vi "Count Encoder Advanced.vi"(6 "Initialise":bool, 7 "Filter Iterations":i16=2, 9 "Encoder B Signal In":bool, 10 "Encoder A Signal In":bool) -> (1 "dt (uS)":i64, 2 "Encoder Count Out":i64)   [LabVIEW 2014]
uses:
  <vilib>/rvi/Emulation/niFpgaGetClockAttributes.vi
  <vilib>/rvi/Emulation/niFpgaSctlEmulationGetInTimedLoop.vi
  <vilib>/rvi/Emulation/niFpgaEmulationReportErrorSimple.vi
  <vilib>/rvi/Emulation/niFpgaCriticalErrorInLSC.vi
panel:
  # "Inputs"
  # "Outputs"
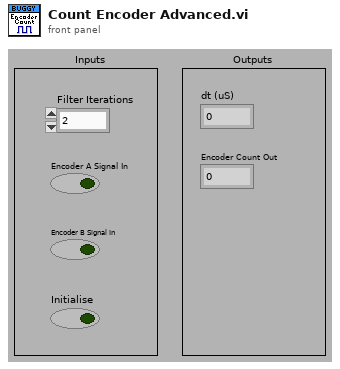
[diagram p1: front panel]
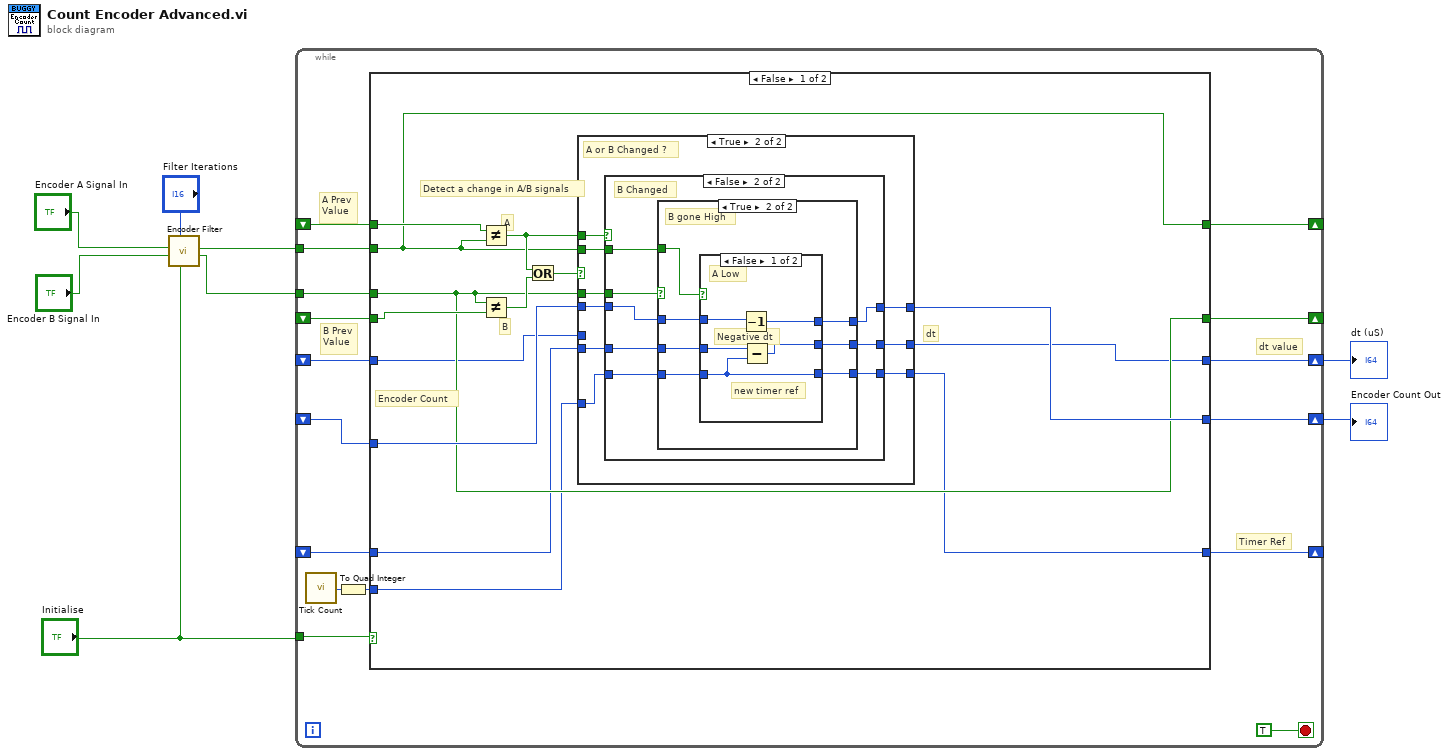
[diagram p0: block diagram]
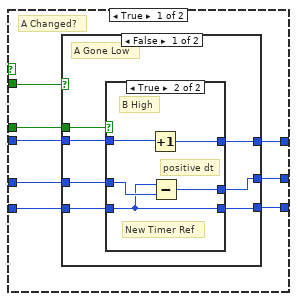
[diagram p3: hidden frame]
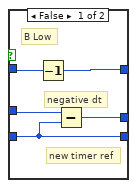
[diagram p4: hidden frame]
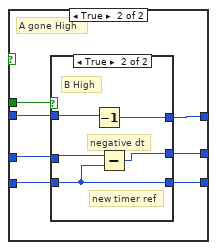
[diagram p5: hidden frame]
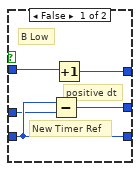
[diagram p6: hidden frame]
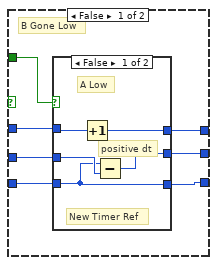
[diagram p7: hidden frame]
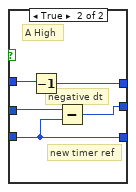
[diagram p8: hidden frame]
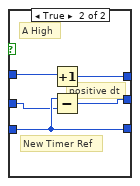
[diagram p9: hidden frame]
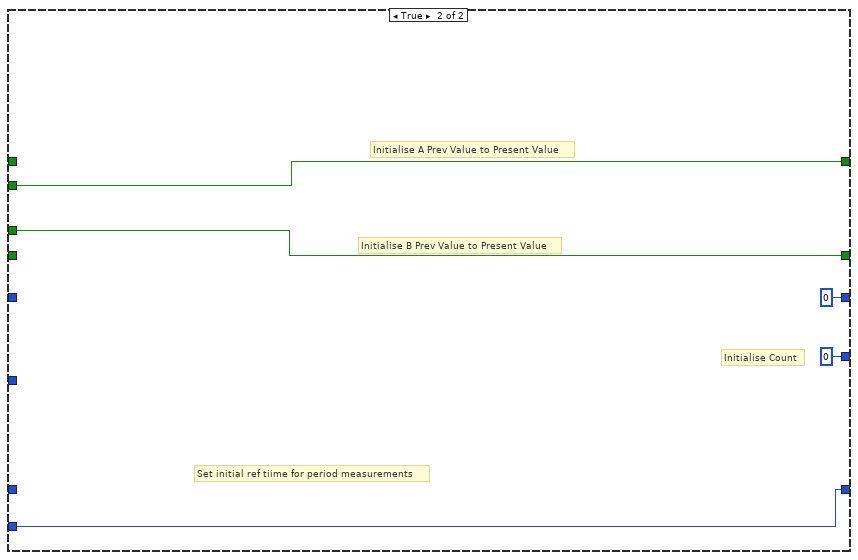
[diagram p10: hidden frame]
diagram:
  n1 = call "Encoder Filter.vi"("Initialise"="Initialise", "Filter Iterations"="Filter Iterations", "Pulse B"="Encoder B Signal In", "Pulse A"="Encoder A Signal In") -> ("Filtered Pulse B"=w4:bool, "Filtered Pulse A"=w5:bool)  [unwired: 6 in]
  n2 = while {
    shift-right: [w22] -> _
    shift-left: _ -> [w17]
    shift-right: [w20] -> _
    shift-left: _ -> [w21]
    tunnel: "Initialise" -> [w15]
    tunnel: w4 -> [w19]
    tunnel: w5 -> [w18]
    shift-right: [w23] -> w8
    shift-left: _ -> [w24]
    shift-right: [w14] -> _
    shift-left: _ -> [w13]
    shift-right: [w12] -> w1
    shift-left: _ -> [w11]
    stop <- TRUE stop-if-true
    # "dt value"
    # "Timer Ref"
    # "B Prev\nValue"
    # "A Prev\nValue"
    n3 = call "Tick Count"() -> ("Tick Count(uSec)"=w10:u32)
    n4 = To Quad Integer(1:w10) -> (0:w9:i64)
    n5 = case shown="False" w15 {
      tunnel: w24 -> [w35 _]
      tunnel: [w34 i64 0] -> w23
      tunnel: [w31 w139] -> w22
      tunnel: w21 -> [w33 _]
      tunnel: [w30 w138] -> w20
      tunnel: w19 -> [w30 w138]
      tunnel: w18 -> [w31 w139]
      tunnel: w17 -> [w32 _]
      tunnel: [w28 w135] -> w14
      tunnel: w13 -> [w29 _]
      tunnel: [w27 i64 0] -> w12
      tunnel: w11 -> [w26 _]
      tunnel: w9 -> [w25 w135]
      frame False {
        # "dt"
        # "Encoder Count"
        # "B"
        # "A"
        # "Detect a change in A/B signals"
        n6 = Not Equal?(x=w32, y=w31) -> (x != y?=w38:bool)
        n7 = Not Equal?(x=w30, y=w33) -> (x != y?=w37:bool)
        n8 = Or(x=w38, y=w37) -> (x .or. y?=w36:bool)
        n9 = case shown="True" w36 {
          tunnel: w38 -> [_ w50]
          tunnel: w35 -> [w41 w49]
          tunnel: w31 -> [_ w48]
          tunnel: w30 -> [_ w47]
          tunnel: [w41 w46] -> w34
          tunnel: w29 -> [w40 w45]
          tunnel: [w40 w43] -> w28
          tunnel: w25 -> [_ w44]
          tunnel: [w39 w42] -> w27
          tunnel: w26 -> [w39 _]
          frame False {
            # "Keep same dt"
            # "Keep same timer ref no pulse hve changed"
            # "A or B not changed Keep Existing encoder count"
          }
          frame True {
            # "A or B Changed ?"
            n10 = case shown="False" w50 {
              tunnel: w49 -> [w58 w100]
              tunnel: w47 -> [w57 w99]
              tunnel: w48 -> [w56 w98]
              tunnel: [w55 w97] -> w46
              tunnel: w45 -> [w54 w96]
              tunnel: w44 -> [w53 w95]
              tunnel: [w52 w93] -> w43
              tunnel: [w51 w94] -> w42
              frame True {
                # "A Changed?"
                n11 = case shown="False" w56 {
                  tunnel: w58 -> [w64 w81]
                  tunnel: w57 -> [w65 w82]
                  tunnel: [w63 w80] -> w55
                  tunnel: w54 -> [w62 w77]
                  tunnel: w53 -> [w60 w79]
                  tunnel: [w59 w78] -> w52
                  tunnel: [w61 w76] -> w51
                  frame False {
                    # "A Gone Low"
                    n12 = case shown="True" w65 {
                      tunnel: w64 -> [w70 w75]
                      tunnel: [w69 w74] -> w63
                      tunnel: w62 -> [w68 w72]
                      tunnel: [w67 w73] -> w61
                      tunnel: w60 -> [w66 w71]
                      tunnel: [w66 w71] -> w59
                      frame False {
                        # "new timer ref"
                        # "negative dt"
                        # "B Low"
                        n13 = Decrement(x=w70) -> (x-1=w69:i64)
                        n14 = Subtract(x=w68, y=w66) -> (x-y=w67:i64)
                      }
                      frame True {
                        # "positive dt"
                        # "New Timer Ref"
                        # "B High"
                        n15 = Increment(x=w75) -> (x+1=w74:i64)
                        n16 = Subtract(x=w71, y=w72) -> (x-y=w73:i64)
                      }
                    }
                  }
                  frame True {
                    # "A gone High"
                    n17 = case shown="True" w82 {
                      tunnel: w81 -> [w86 w92]
                      tunnel: [w87 w91] -> w80
                      tunnel: w79 -> [w85 w89]
                      tunnel: [w85 w89] -> w78
                      tunnel: w77 -> [w84 w90]
                      tunnel: [w83 w88] -> w76
                      frame False {
                        # "positive dt"
                        # "New Timer Ref"
                        # "B Low"
                        n18 = Subtract(x=w85, y=w84) -> (x-y=w83:i64)
                        n19 = Increment(x=w86) -> (x+1=w87:i64)
                      }
                      frame True {
                        # "new timer ref"
                        # "negative dt"
                        # "B High"
                        n20 = Decrement(x=w92) -> (x-1=w91:i64)
                        n21 = Subtract(x=w90, y=w89) -> (x-y=w88:i64)
                      }
                    }
                  }
                }
              }
              frame False {
                # "B Changed"
                n22 = case shown="True" w99 {
                  tunnel: w100 -> [w107 w124]
                  tunnel: [w106 w123] -> w97
                  tunnel: w98 -> [w105 w122]
                  tunnel: w96 -> [w104 w121]
                  tunnel: w95 -> [w103 w120]
                  tunnel: [w102 w119] -> w94
                  tunnel: [w101 w118] -> w93
                  frame False {
                    # "B Gone Low"
                    n23 = case shown="False" w105 {
                      tunnel: w107 -> [w112 w117]
                      tunnel: [w111 w116] -> w106
                      tunnel: w104 -> [w110 w113]
                      tunnel: w103 -> [w108 w115]
                      tunnel: [w109 w114] -> w102
                      tunnel: [w108 w115] -> w101
                      frame False {
                        # "positive dt"
                        # "New Timer Ref"
                        # "A Low"
                        n24 = Increment(x=w112) -> (x+1=w111:i64)
                        n25 = Subtract(x=w108, y=w110) -> (x-y=w109:i64)
                      }
                      frame True {
                        # "new timer ref"
                        # "negative dt"
                        # "A High"
                        n26 = Decrement(x=w117) -> (x-1=w116:i64)
                        n27 = Subtract(x=w113, y=w115) -> (x-y=w114:i64)
                      }
                    }
                  }
                  frame True {
                    # "B gone High"
                    n28 = case shown="False" w122 {
                      tunnel: w124 -> [w129 w134]
                      tunnel: [w128 w133] -> w123
                      tunnel: w121 -> [w127 w131]
                      tunnel: w120 -> [w126 w132]
                      tunnel: [w125 w130] -> w119
                      tunnel: [w126 w132] -> w118
                      frame False {
                        # "new timer ref"
                        # "Negative dt"
                        # "A Low"
                        n29 = Decrement(x=w129) -> (x-1=w128:i64)
                        n30 = Subtract(x=w127, y=w126) -> (x-y=w125:i64)
                      }
                      frame True {
                        # "positive dt"
                        # "New Timer Ref"
                        # "A High"
                        n31 = Increment(x=w134) -> (x+1=w133:i64)
                        n32 = Subtract(x=w132, y=w131) -> (x-y=w130:i64)
                      }
                    }
                  }
                }
              }
            }
          }
        }
      }
      frame True {
        # "Set initial ref tiime for period measurements"
        # "Initialise Count"
        # "Initialise B Prev Value to Present Value"
        # "Initialise A Prev Value to Present Value"
      }
    }
  }
  "Encoder Count Out" <- w8
  "dt (uS)" <- w1
